vi "Progress Bar Controller.vi"(0 "Action":T1, 5 "Slide":refnum<vi>, 7 "Caption.Text":string="Running script", 11 "error in (no error)":errorcluster) -> (15 "error out":errorcluster)   [LabVIEW 2020]
uses:
  PBar-Action.ctl
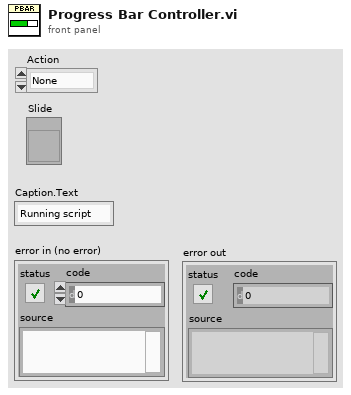
[diagram p1: front panel]
types:
  T1 = typedef "PBar-Action.ctl" = enum16{"None", "Start", "Clear"}
  T2 = enum32{"Invalid", "Standard", "Closed", "Hidden", "Minimized", "Maximized"}
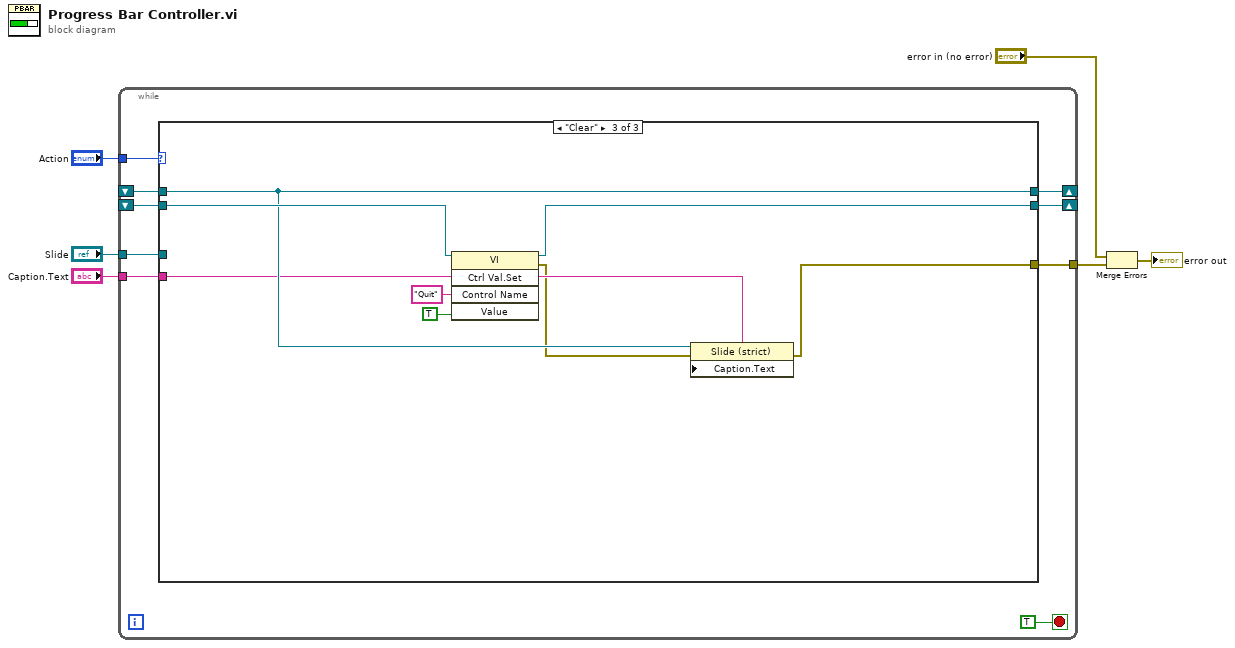
[diagram p0: block diagram]
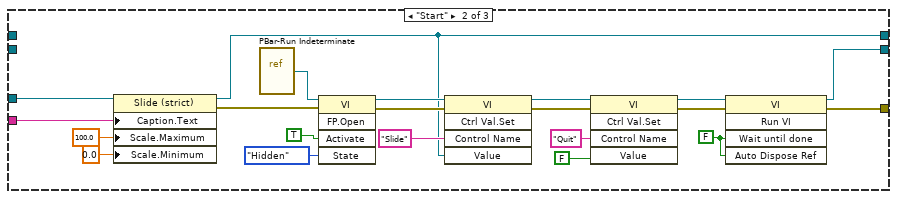
[diagram p3: hidden frame]
diagram:
  n1 = while {
    tunnel: "Action" -> [w15]
    shift-right: [w12] -> _
    shift-left: _ -> [w14]
    tunnel: "Caption.Text" -> [w13]
    shift-right: [w11] -> _
    shift-left: _ -> [w10]
    tunnel: "Slide" -> [w9]
    tunnel: [w7] -> w3
    stop <- TRUE stop-if-true
    n2 = case shown="\"Clear\"" w15 {
      tunnel: w14 -> [w17 _ w42]
      tunnel: w13 -> [_ w22 w41]
      tunnel: [w17 w19 w42] -> w12
      tunnel: [w16 w21 w43] -> w11
      tunnel: w10 -> [w16 _ w44]
      tunnel: w9 -> [_ w20 _]
      tunnel: [_ w18 w39] -> w7
      frame "None", Default {
      }
      frame "Start" {
        w37 = FALSE ("Wait Until Done")
        n3 = property class="Slide (strict)"(reference=w20, "Caption.Text"=w22, "Scale.Maximum"=100.0 ("y"), "Scale.Minimum"=0.0 ("Scale.Range:Minimum")) -> (reference out=w19:refnum<vi>, error out=w33:errorcluster)  [unwired: 1 in]
        n4 = vi-ref "PBar-Run Indeterminate.vi"() -> (w35:refnum<vi>)
        n5 = invoke class="VI" method="FP.Open"(reference=w35, error in=w33, "Activate"=TRUE ("Activate?"), "State"=T2."Hidden") -> (reference out=w32:refnum<vi>, error out=w31:errorcluster)  [unwired: 1 in, 3 out]
        n6 = invoke class="VI" method="Ctrl Val.Set"(reference=w32, error in=w31, "Control Name"="Slide", "Value"=w19) -> (reference out=w28:refnum<vi>, error out=w27:errorcluster)  [unwired: 1 in, 3 out]
        n7 = invoke class="VI" method="Ctrl Val.Set"(reference=w28, error in=w27, "Control Name"="Quit", "Value"=FALSE) -> (reference out=w26:refnum<vi>, error out=w25:errorcluster)  [unwired: 1 in, 3 out]
        n8 = invoke class="VI" method="Run VI"(reference=w26, error in=w25, "Wait until done"=w37, "Auto Dispose Ref"=w37) -> (reference out=w21:refnum<vi>, error out=w18:errorcluster)  [unwired: 1 in, 3 out]
      }
      frame "Clear" {
        n9 = invoke class="VI" method="Ctrl Val.Set"(reference=w44, "Control Name"="Quit", "Value"=TRUE) -> (reference out=w43:refnum<vi>, error out=w40:errorcluster)  [unwired: 2 in, 3 out]
        n10 = property class="Slide (strict)"(reference=w42, error in=w40, "Caption.Text"=w41) -> (error out=w39:errorcluster)  [unwired: 1 out]
      }
    }
  }
  n11 = Merge Errors("error in (no error)", w3) -> (→"error out":errorcluster)
